vi "DeBounce_Error.vi"(8 "error in (no error)":errorcluster) -> (0 "error out":errorcluster)   [LabVIEW 2018]
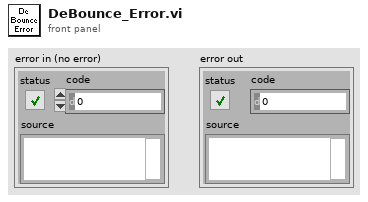
[diagram p1: front panel]
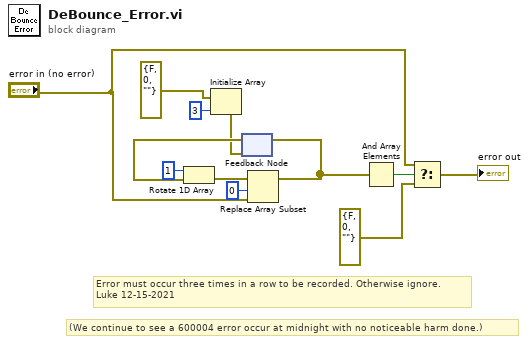
[diagram p0: block diagram]
diagram:
  # "(We continue to see a 600004 error occur at midnight with no noticeable harm done.)"
  # "Error must occur three times in a row to be recorded. Otherwise ignore.\nLuke 12-15-2021"
  n1 = Initialize Array(errorcluster {"status"=FALSE, "code"=0, "source"=""} ("error in (no error)"), 3 ("dimension size")) -> (w4:errorcluster[])
  n2 = feedback #1(w4) -> (w12:errorcluster[])
  n3 = Rotate 1D Array(1:w12, 2:1 ("n")) -> (0:w11:errorcluster[])
  n4 = Replace Array Subset(array=w11, new element="error in (no error)", index=0) -> (w9:errorcluster[])
  n5 = feedback-in #1(w9) -> ()
  n6 = And Array Elements(Boolean array=w9) -> (logical AND=w5:bool)
  n7 = Select(t="error in (no error)", s=w5, f=errorcluster {"status"=FALSE, "code"=0, "source"=""}) -> (s? t:f=→"error out":errorcluster)
